vi "Send status.vi"(8 "error in (no error)":errorcluster, 11 "Channel in":refnum<class "Channel.lvclass">) -> (0 "error out":errorcluster, 3 "Channel out":refnum<class "Channel.lvclass">)   [LabVIEW 2018, in "Channel.lvclass"]
uses:
  Channel.lvclass
  Channel.lvclass/Channel.ctl
  Simulated_CCD_Camera/Simulated_CCD_Camera.lvclass/Simulated_CCD_Camera.ctl
  Simulated_CCD_Camera/Simulated_CCD_Camera.lvclass
  RxTx/RxTx.lvclass
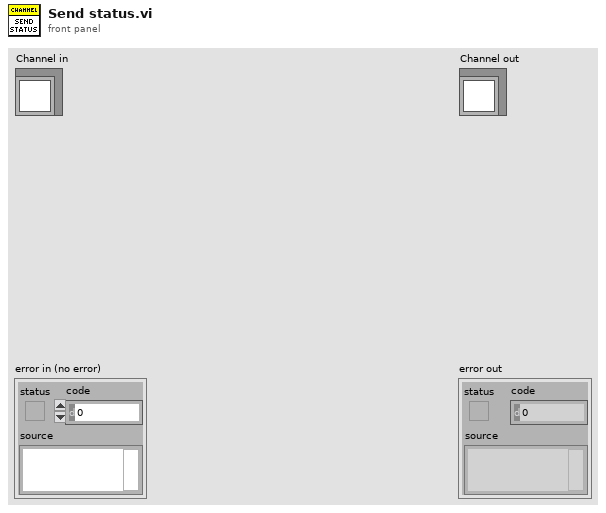
[diagram p1: front panel]
types:
  T1 = cluster{"CYCLES_DONE":u16, "LAST_IMAGE_NAME":string, "DISK_SPACE":u16, "FRAMES_DONE":u16, "CCD_STATUS":string, "CURRENT_TEMPERATURE":i16, "TEMPERATURE_STATUS":string, "FRAME_EXPOSURE_TIME":sgl, "ERROR":bool, "SERIAL_NUMBER":u16, "ACQUIRING":bool, "IMAGE_INDEX":u32, "SEQS_DONE":u16}
  T2 = cluster{"PREAMP":u16, "READOUT_RATE":u16, "EM_GAIN":u16, "VERTICAL_SHIFT_SPEED":u16, "READ_MODE":u16, "FRAME_TRANSFER":bool, "VERTICAL_CLOCK_VOLTAGE":u16, "ACQUISITION_MODE":u16, "AD_CHANNEL":u16, "EM_MODE":u16, "SHUTTER_TTL":u16, "SHUTTER_OPENING_TIME":u16, "SHUTTER_CLOSING_TIME":u16, "SHUTTER_MODE":u16, "TRIGGER_MODE":u16, "VBIN":u16, "INITIAL_LINE":u16, "INITIAL_COLUMN":u16, "FINAL_LINE":u16, "FINAL_COLUMN":u16, "HBIN":u16}
  T3 = cluster{"COOLER_POWER_STATUS":u16, "TEMP":i32, "EXPTIME":dbl, "#FRAMES":u32, "#CYCLES":u32, "#SEQS":u32, "WAVEPLATE_POS":u16}
  T4 = cluster{"CCD status":string, "CCD configuration":string, "Acquisition configuration":string}
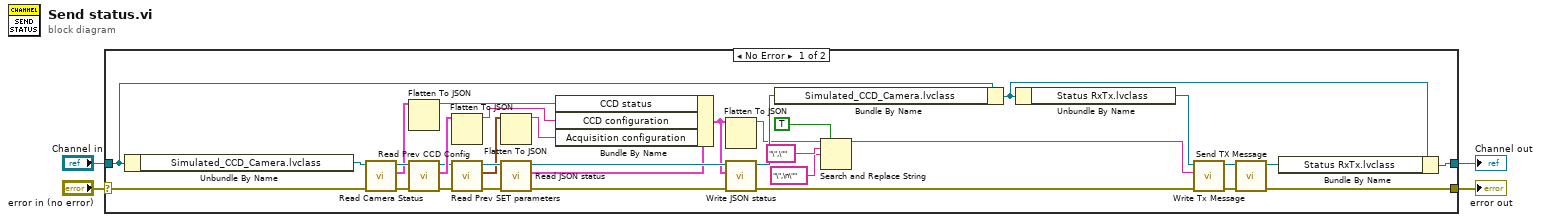
[diagram p0: block diagram]
diagram:
  n1 = case shown="No Error" "error in (no error)" {
    selector: "error in (no error)" -> [w20 w39]
    tunnel: [w32 w39] -> w3
    tunnel: [w31 w38] -> w1
    tunnel: "Channel in" -> [w30 w38]
    frame No Error {
      n2 = Unbundle By Name(w30) -> ("Simulated_CCD_Camera.lvclass"=w21:refnum<class "Simulated_CCD_Camera.lvclass">)
      n3 = call "Read Camera Status.vi"("error in (no error)"=w20, "CCDCamera in"=w21) -> ("error out"=w19:errorcluster, "Camera Status"=w17:T1, "CCDCamera out"=w22:refnum<class "Simulated_CCD_Camera.lvclass">)  [unwired: 7 in]
      n4 = Flatten To JSON(anything=w17) -> (JSON string=w18:string)  [unwired: 2 in, 1 out]
      n5 = call-dynamic "Read Prev CCD Config.vi"("error in (no error)"=w19, "Simulated_CCD_Camera in"=w22) -> ("error out"=w15:errorcluster, "Prev CCD Config"=w26:T2, "Simulated_CCD_Camera out"=w16:refnum<class "Simulated_CCD_Camera.lvclass">)  [unwired: 7 in]
      n6 = Flatten To JSON(anything=w26) -> (JSON string=w27:string)  [unwired: 2 in, 1 out]
      n7 = call-dynamic "Read Prev SET parameters.vi"("error in (no error)"=w15, "Simulated_CCD_Camera in"=w16) -> ("error out"=w14:errorcluster, "Prev SET parameters"=w12:T3, "Simulated_CCD_Camera out"=w13:refnum<class "Simulated_CCD_Camera.lvclass">)  [unwired: 7 in]
      n8 = Flatten To JSON(anything=w12) -> (JSON string=w11:string)  [unwired: 2 in, 1 out]
      n9 = call "Read JSON status.vi"("error in (no error)"=w14, "Simulated_CCD_Camera in"=w13) -> ("error out"=w28:errorcluster, "JSON status"=w6:T4, "Simulated_CCD_Camera out"=w29:refnum<class "Simulated_CCD_Camera.lvclass">)  [unwired: 7 in]
      n10 = Bundle By Name(cluster=w6, "CCD status"=w18, "CCD configuration"=w27, "Acquisition configuration"=w11) -> (w23:T4)
      n11 = Flatten To JSON(anything=w23) -> (JSON string=w10:string)  [unwired: 2 in, 1 out]
      n12 = call "Write JSON status.vi"("error in (no error)"=w28, "JSON status"=w23, "Simulated_CCD_Camera in"=w29) -> ("error out"=w24:errorcluster, "Simulated_CCD_Camera out"=w25:refnum<class "Simulated_CCD_Camera.lvclass">)  [unwired: 7 in]
      n13 = Bundle By Name(cluster=w30, "Simulated_CCD_Camera.lvclass"=w25) -> (w37:refnum<class "Channel.lvclass">)
      n14 = Search and Replace String(replace all?=TRUE ("replace all? (F)"), input string=w10, search string="\",\"", replace string="\",\n\"" ("search string")) -> (result string=w5:string)  [unwired: 4 in, 3 out]
      n15 = Unbundle By Name(w37) -> ("Status RxTx.lvclass"=w33:refnum<class "RxTx.lvclass">)
      n16 = call "Write Tx Message.vi"("error in (no error)"=w24, "Tx Message"=w5, "RxTx in"=w33) -> ("error out"=w34:errorcluster, "RxTx out"=w36:refnum<class "RxTx.lvclass">)  [unwired: 7 in]
      n17 = call "Send TX Message.vi"("error in (no error)"=w34, "RxTx in"=w36) -> ("error out"=w32:errorcluster, "RxTx out"=w35:refnum<class "RxTx.lvclass">)  [unwired: 8 in]
      n18 = Bundle By Name(cluster=w37, "Status RxTx.lvclass"=w35) -> (w31:refnum<class "Channel.lvclass">)
    }
    frame Error {
    }
  }
  "error out" <- w3
  "Channel out" <- w1
